vi "write.vi"(6 "写入缓冲区":string, 7 "写入缓冲区 2":string, 9 "布尔":bool, 10 "VISA资源名称输入":refnum<visa-resource-name>, 11 "VISA引用句柄输入":refnum<visa-resource-name>) -> ()   [LabVIEW 2016]
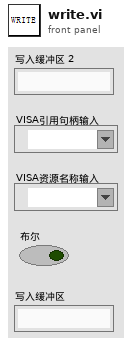
[diagram p1: front panel]
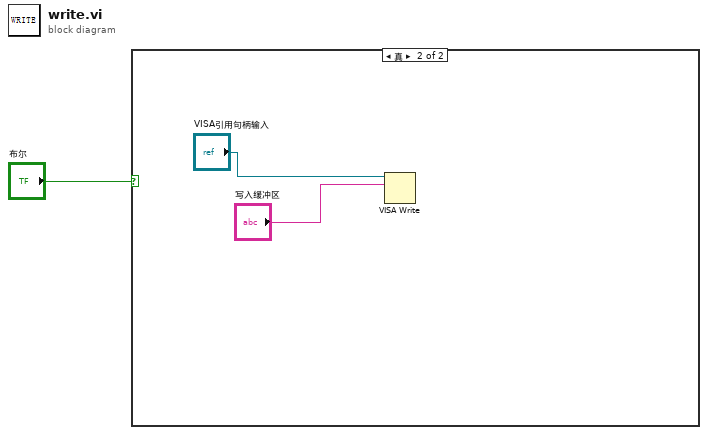
[diagram p0: block diagram]
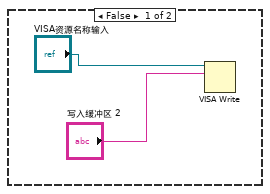
[diagram p2: hidden frame]
diagram:
  n1 = case shown="真" "布尔" {
    frame False {
      n2 = VISA Write(VISA resource name="VISA资源名称输入", write buffer="写入缓冲区 2") -> ()  [unwired: 1 in, 3 out]
    }
    frame True {
      n3 = VISA Write(VISA resource name="VISA引用句柄输入", write buffer="写入缓冲区") -> ()  [unwired: 1 in, 3 out]
    }
  }
